vi "Format TXP.vi"(10 "TxP Results":T1) -> (2 "Txp Results":T2)   [LabVIEW 2015, in "niDTS BT.lvlib" / "niDTS BT INSTR TX.lvclass"]
uses:
  niDTS BT INSTR TX.lvclass
  Tests/Tx Test/Includes/niDTS BT Tx Test INC TXP Results.ctl
  niDTS BT.lvlib
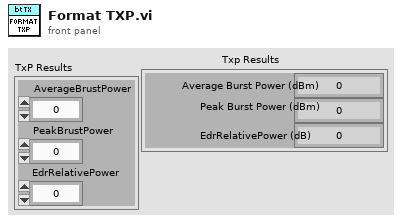
[diagram p1: front panel]
types:
  T1 = cluster{"AverageBrustPower":dbl, "PeakBrustPower":dbl, "EdrRelativePower":dbl}
  T2 = typedef "niDTS BT.lvlib/niDTS BT Tx Test INC TXP Results.ctl" = cluster{"Average Burst Power (dBm)":dbl, "Peak Burst Power (dBm)":dbl, "EdrRelativePower (dB)":dbl}
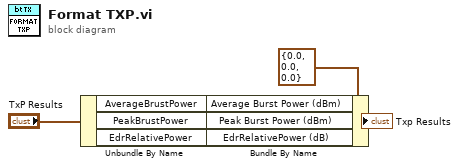
[diagram p0: block diagram]
diagram:
  n1 = Unbundle By Name("TxP Results") -> ("AverageBrustPower"=w5:dbl, "PeakBrustPower"=w4:dbl, "EdrRelativePower"=w1:dbl)
  n2 = Bundle By Name(cluster=T2 {"Average Burst Power (dBm)"=0.0, "Peak Burst Power (dBm)"=0.0, "EdrRelativePower (dB)"=0.0} ("TXP Resutls"), "Average Burst Power (dBm)"=w5, "Peak Burst Power (dBm)"=w4, "EdrRelativePower (dB)"=w1) -> (→"Txp Results":T2)
